vi "New.vi"(9 "Baud rate (38400)":u32=38400, 10 "Terminator (CR)":u8=13 format="%x", 11 "VISA resource name":refnum<visa-resource-name>) -> (0 "error out":errorcluster, 3 "Serial Device out":refnum<class "Serial Device.lvclass">)   [LabVIEW 2015, in "Serial Device.lvclass"]
uses:
  Serial Device.lvclass
  Serial Device.lvclass/Serial Device.ctl
  <vilib>/Instr/_visa.llb/VISA Configure Serial Port (Instr).vi
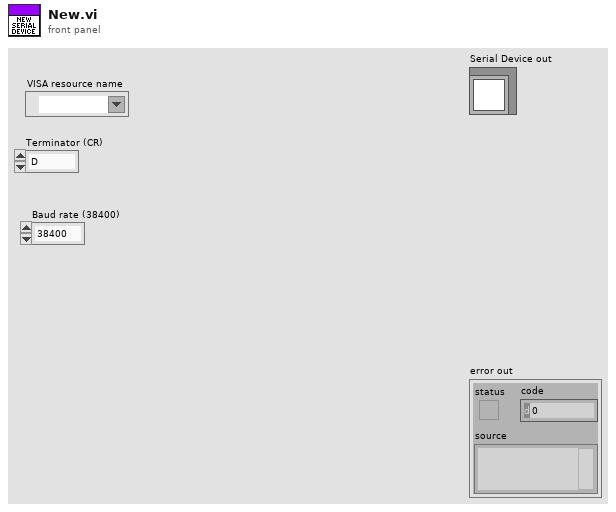
[diagram p1: front panel]
types:
  T1 = typedef "Semaphore RefNum" = refnum<k1>
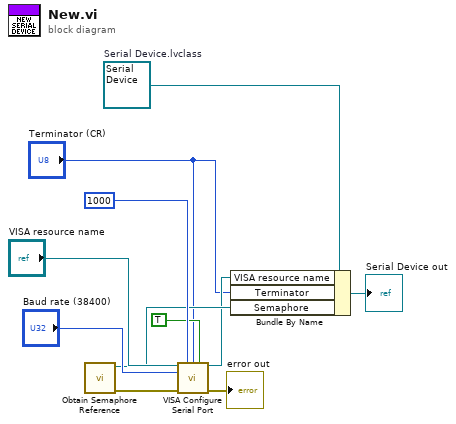
[diagram p0: block diagram]
diagram:
  w11 = refnum<class "Serial Device.lvclass"> refnum  # Serial Device.lvclass
  n1 = call <vilib>:"Obtain Semaphore Reference.vi"() -> ("error out"=w6:errorcluster, "semaphore"=w4:T1)  [unwired: 5 in, 1 out]
  n2 = call-poly "VISA Configure Serial Port"("VISA resource name"="VISA resource name", "timeout (10sec)"=u32 1000, "termination char\n(0xA = '\\n' = LF)"="Terminator (CR)", "Enable Termination\nChar (T)"=TRUE ("Enable Termination\nChar (T)"), "baud rate (9600)"="Baud rate (38400)", "error in (no error)"=w6) -> ("VISA resource name out"=w3:refnum<visa-resource-name>, "error out"=→"error out":errorcluster)  [unwired: 8 in]
  n3 = Bundle By Name(cluster=w11, "VISA resource name"=w3, "Terminator"="Terminator (CR)", "Semaphore"=w4) -> (→"Serial Device out":refnum<class "Serial Device.lvclass">)
